vi "Stop Core.vi"(10 "final error code":i32, 11 "Preparation Line in":refnum<class "Preparation Line.lvclass">) -> (3 "Preparation Line out":refnum<class "Preparation Line.lvclass">)   [LabVIEW 2015, in "cRIO-Carbondioxide.lvlib" / "CO2-Actor.lvlib" / "Preparation Line.lvclass"]
doc: "(<B>Filename</B>: Actor Framework.lvlib:Actor.lvclass:Stop Core.vi)\n\nDefines what the actor does before it stops. Use the <B>final error code</B> input to determine whether the actor shut down in response to an error.\n\nBy default, this method does nothing. A descendant class may override it to define behavior, such as shutting down any processes the actor initiated in its override of the Actor Core method."
uses:
  Preparation Line.lvclass
  Preparation Line.lvclass/Preparation Line.ctl
  CO2 Actor/CO2 Actor.lvclass
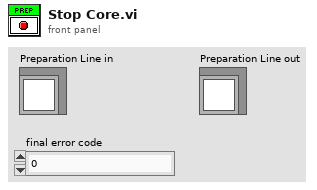
[diagram p1: front panel]
types:
  T1 = typedef "Sample Container.ctl" = cluster{"Sample In":refnum<k21>, "Sample Name":refnum<k21>, "Ti Cathode":refnum<k21>, "SampleQ":refnum<queue>}
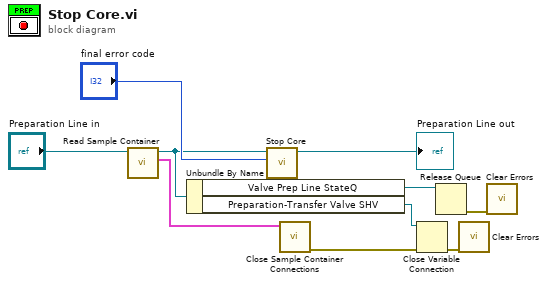
[diagram p0: block diagram]
diagram:
  n1 = call "Read Sample Container.vi"("Preparation Line in"="Preparation Line in") -> ("Container"=w7:T1, "Preparation Line out"=w6:refnum<class "Preparation Line.lvclass">)  [unwired: 7 in, 2 out]
  n2 = Unbundle By Name(w6) -> ("Valve Prep Line StateQ"=w2:refnum<queue>, "Preparation-Transfer Valve SHV"=w5:refnum<k21>)
  n3 = call-parent "Stop Core.vi"("final error code"="final error code", "CO2 Actor in"=w6) -> ("CO2 Actor out"=→"Preparation Line out":refnum<class "Preparation Line.lvclass">)  [unwired: 9 in]
  n4 = call "Close Sample Container Connections.vi"("Container in"=w7) -> ("error out"=w4:errorcluster)  [unwired: 9 in, 1 out]
  n5 = Close Variable Connection(8:w4, 11:w5) -> (0:w3:errorcluster)
  n6 = Release Queue(queue=w2) -> (error out=w1:errorcluster)  [unwired: 2 in, 2 out]
  n7 = call <vilib>:"Clear Errors.vi"("error in (no error)"=w3) -> ()  [unwired: 5 in, 2 out]
  n8 = call <vilib>:"Clear Errors.vi"("error in (no error)"=w1) -> ()  [unwired: 5 in, 2 out]
